vi "LINC Convert CMD to Readable Text.vi"(6 "command name in":string, 7 "command data in":string, 9 "parameter formats":T1[](array[typedef]), 10 "parameter names":string[](array[string]), 11 "LINC in":refnum<class "LINC.lvclass">) -> (2 "Cmd Text":string, 3 "LINC out":refnum<class "LINC.lvclass">)   [LabVIEW 2018, in "STEPkgDriver_LINC.lvlib" / "LINC.lvclass"]
doc: "Converts the incoming command into readable command text for use in GUIs and logs."
uses:
  LINC.lvclass
  LINC Format Prototype.ctl
  STEPkgDriver_LINC.lvlib
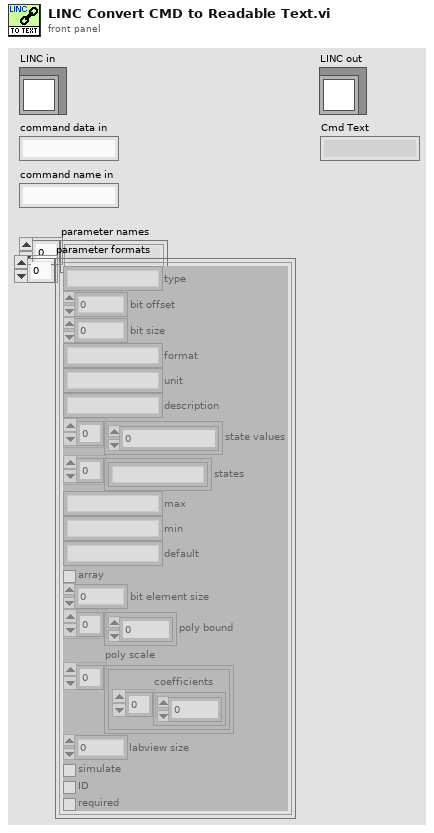
[diagram p1: front panel]
types:
  T1 = typedef "STEPkgDriver_LINC.lvlib/LINC Format Prototype.ctl" = cluster{"type":string, "bit offset":i32, "bit size":i32, "format":string, "unit":string, "description":string, "state values":i64[], "states":string[], "max":string, "min":string, "default":string, "array":bool, "bit element size":i32, "poly bound":dbl[], "poly scale":cluster{"coefficients":dbl[]}[], "labview size":i32, "simulate":bool, "ID":bool, "required":bool}
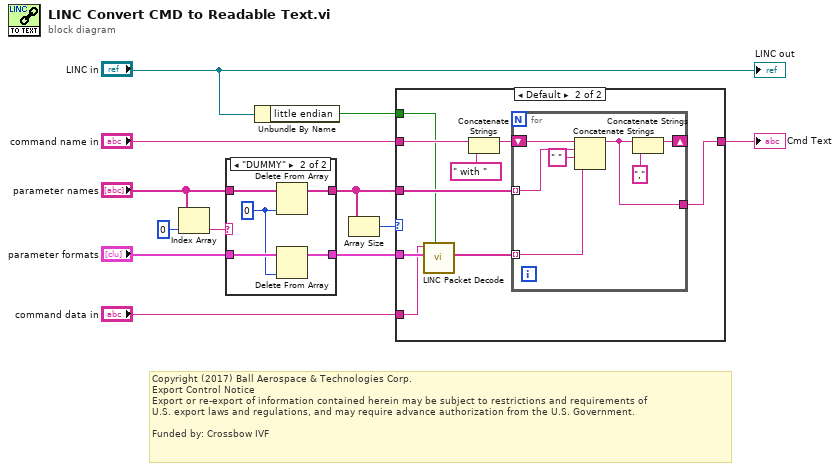
[diagram p0: block diagram]
diagram:
  # "Copyright (2017) Ball Aerospace & Technologies Corp. \nExport Control Notice\nExport or re-export of information contained herein may be subject to restrictions and requirements of \nU.S. export laws and regulations, and may require advance authorization from the U.S. Government.\n\nFunded by: Crossbow IVF"
  n1 = Index Array(array="parameter names", index=0) -> (element=w10:string)
  n2 = case shown="\"DUMMY\"" w10 {
    tunnel: "parameter names" -> [w14 w19]
    tunnel: [w14 w18] -> w5
    tunnel: [w13 w17] -> w6
    tunnel: "parameter formats" -> [w13 w16]
    frame Default {
    }
    frame "DUMMY" {
      w15 = 0 ("index")
      n3 = Delete From Array(array=w19, index=w15) -> (array with subset deleted=w18:string[])  [unwired: 1 in, 1 out]
      n4 = Delete From Array(array=w16, index=w15) -> (array with subset deleted=w17:T1[])  [unwired: 1 in, 1 out]
    }
  }
  n5 = Unbundle By Name("LINC in") -> ("little endian"=w12:bool)
  n6 = Array Size(array=w5) -> (size(s)=w2:i32)
  n7 = case shown="Default" w2 {
    tunnel: "command name in" -> [w20 w27]
    tunnel: [w20 w24] -> w4
    tunnel: w5 -> [_ w25]
    tunnel: w6 -> [_ w23]
    tunnel: w12 -> [_ w22]
    tunnel: "command data in" -> [_ w21]
    frame 0 {
    }
    frame Default {
      n8 = call "LINC Packet Decode.vi"("little endian"=w22, "item formats"=w23, "data in"=w21) -> ("decoded items"=w29:string[])  [unwired: 8 in]
      n9 = Concatenate Strings(w27, " with " ("string")) -> (w28:string)
      n10 = for {
        shift-right: [w32] -> _
        shift-left: w28 -> [w36]
        tunnel: w29 -> [w34] mode=indexing
        tunnel: w25 -> [w35] mode=indexing
        tunnel: [w31] -> w24
        n11 = Concatenate Strings(w36, w35, " " ("string"), w34) -> (w31:string)
        n12 = Concatenate Strings(w31, "," ("string")) -> (w32:string)
      }
    }
  }
  "Cmd Text" <- w4
  "LINC out" <- "LINC in"
